vi "CalcOctaves.vi"(11 "Energy":cluster{"x0":dbl, "df":dbl, dbl[]}[](graph)) -> (1 "XY Graph":cluster{dbl[], dbl[]}[](graph), 2 "Prediction":dbl[](array[numeric]), 3 "Peak Freq":dbl[](array[numeric]))   [LabVIEW 2022 SP3]
uses:
  <vilib>/Analysis/NI_AAL_SigProc.lvlib
panel:
  out "Energy 2":cluster{"x0":dbl, "df":dbl, dbl[]}(graph)
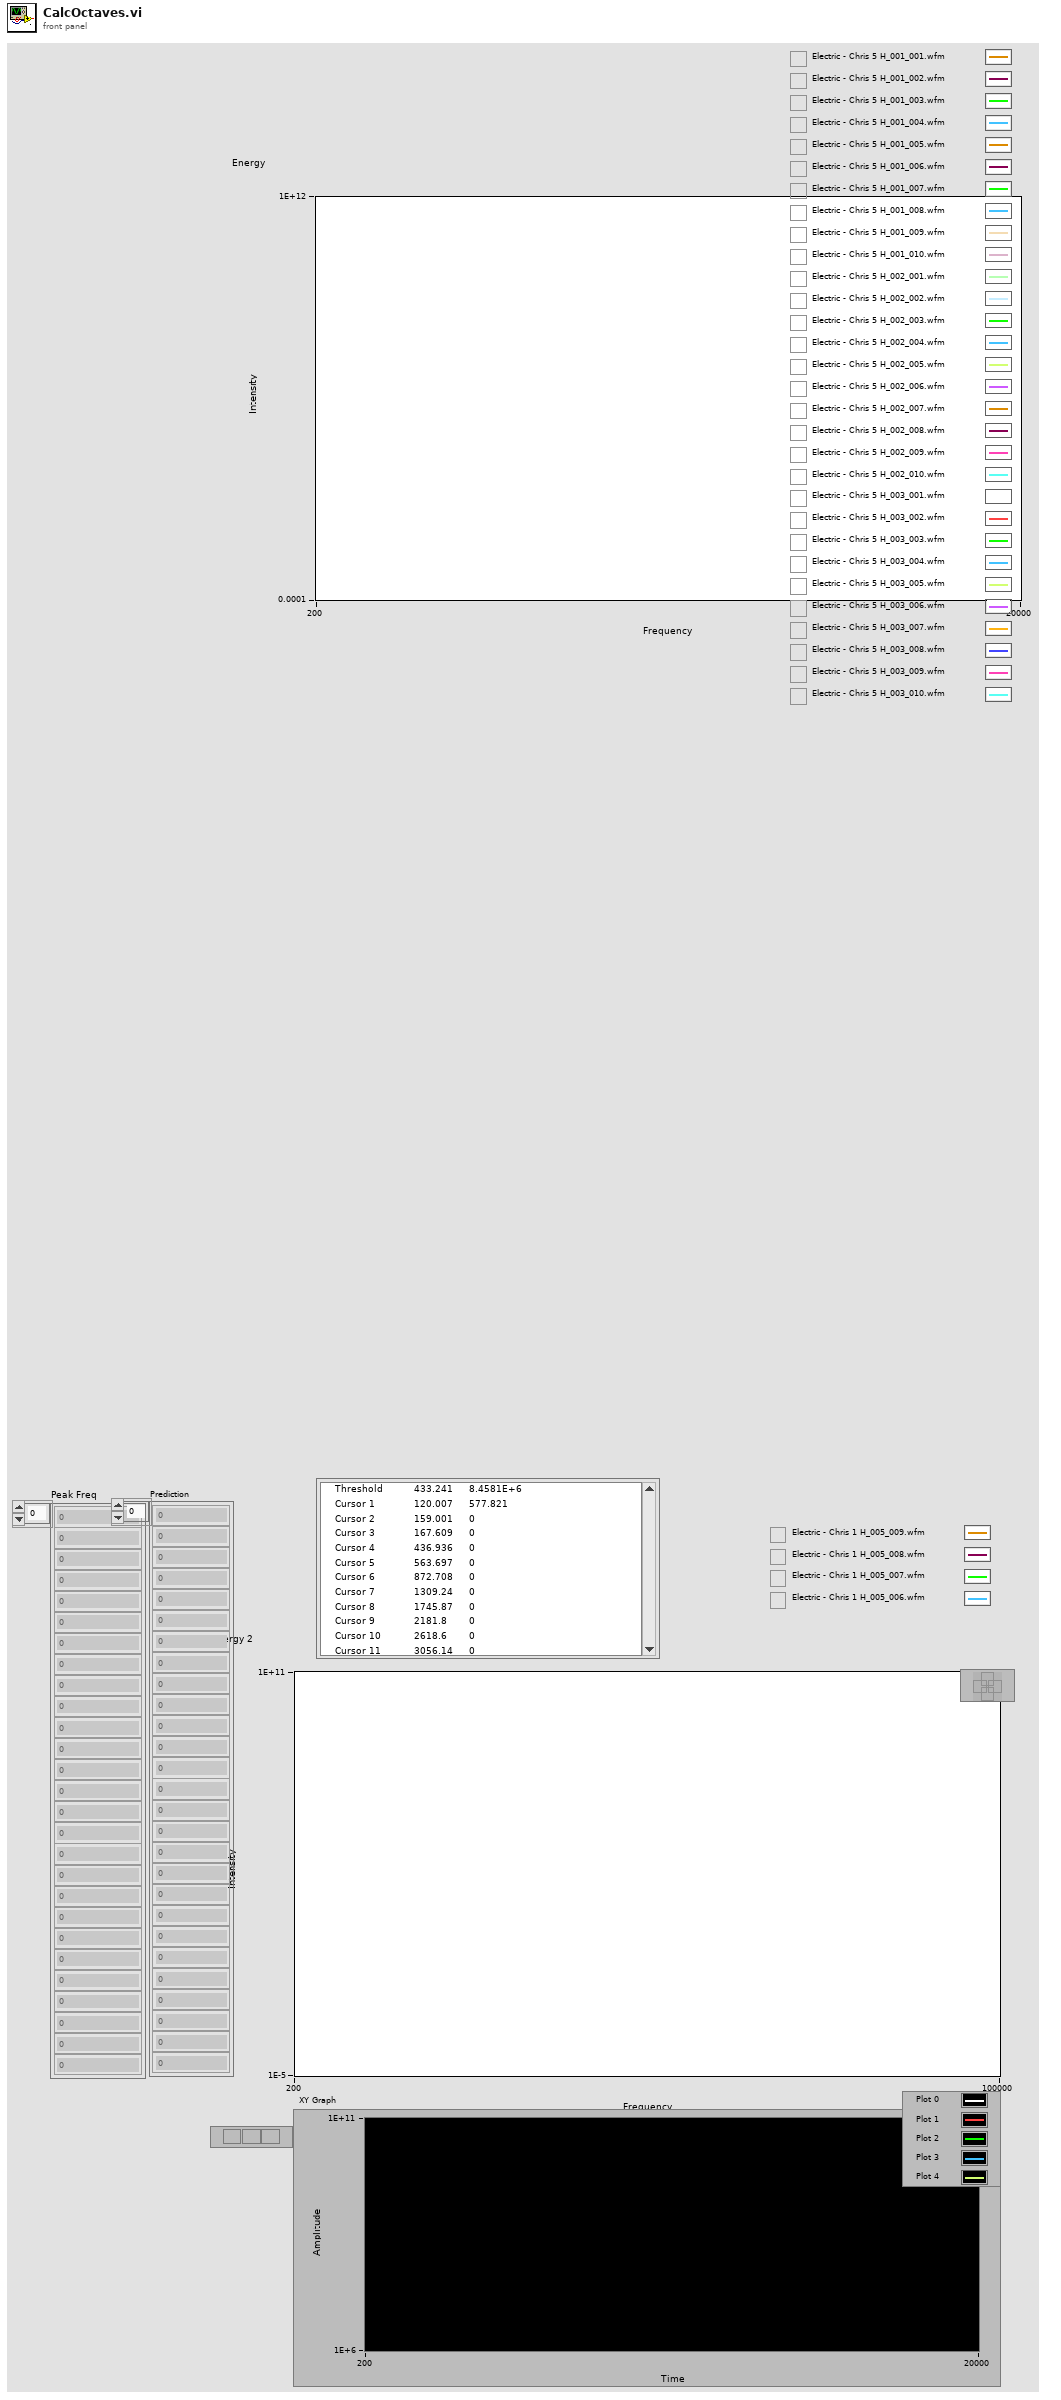
[diagram p1: front panel]
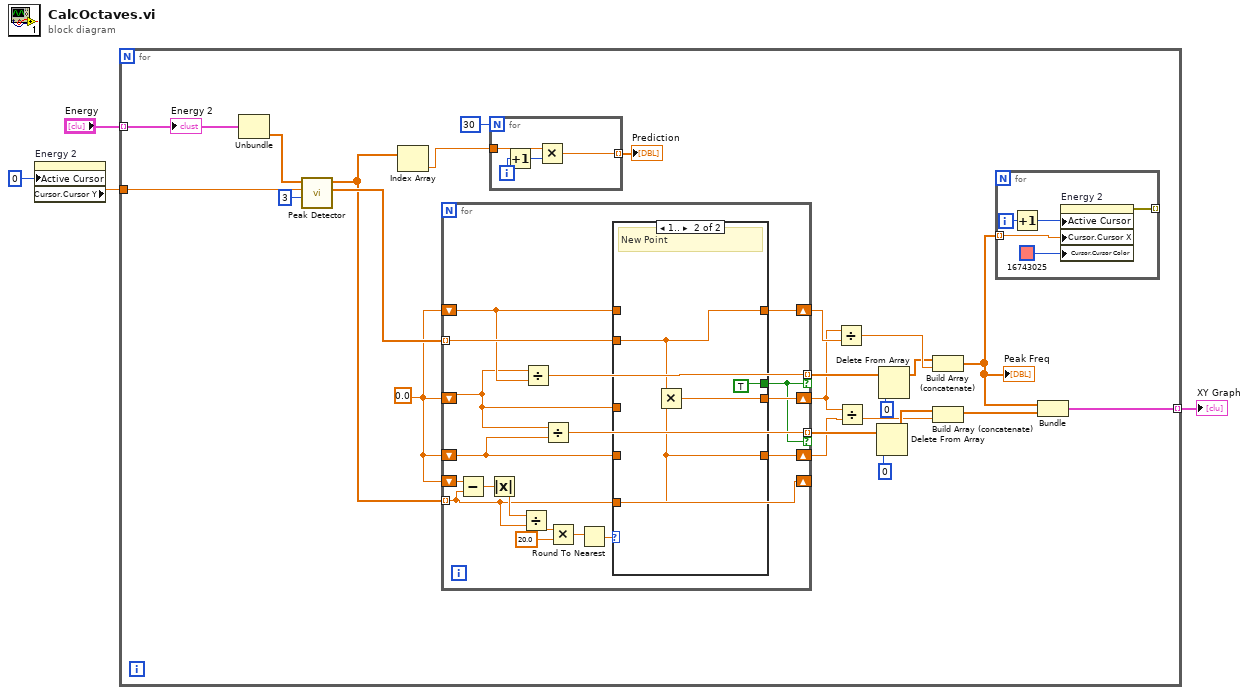
[diagram p0: block diagram]
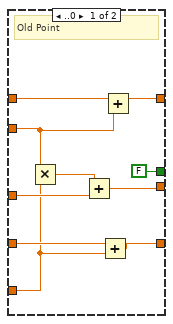
[diagram p2: hidden frame]
diagram:
  n1 = property on="Energy 2" class="WFGraph (strict)"("Active Cursor"=u32 0) -> ("Cursor.Cursor Y"=w3:dbl)  [unwired: 2 in, 2 out]
  n2 = for {
    tunnel: w3 -> [w27]
    tunnel: [w8] -> w2 mode=indexing
    tunnel: "Energy" -> [w5] mode=indexing
    w15 = 0.0
    n3 = Unbundle(w5) -> (w28:dbl[])  [unwired: 2 out]
    n4 = call <vilib>:"Peak Detector.vi"("width"=3, "threshold"=w27, "X"=w28) -> ("Amplitudes"=w24:dbl[], "Locations"=w20:dbl[])  [unwired: 4 in, 3 out]
    n5 = Index Array(array=w20) -> (element=w19:dbl)  [unwired: 1 in]
    n6 = for {
      tunnel: w20 -> [w43] mode=indexing
      shift-right: [w43] -> _
      shift-left: w15 -> [w50]
      shift-right: [w41] -> w12
      shift-left: w15 -> [w36]
      tunnel: [w42] -> w26 mode=indexing if=w33
      shift-right: [w39] -> w23
      shift-left: w15 -> [w38]
      tunnel: w24 -> [w40] mode=indexing
      shift-right: [w37] -> w11
      shift-left: w15 -> [w35]
      tunnel: [w34] -> w13 mode=indexing if=w33
      n7 = Subtract(x=w50, y=w43) -> (x-y=w49:dbl)
      n8 = Absolute Value(x=w49) -> (abs(x)=w48:dbl)
      n9 = Divide(x=w48, y=w43) -> (x/y=w47:dbl)
      n10 = Divide(x=w36, y=w38) -> (x/y=w42:dbl)
      n11 = Divide(x=w36, y=w35) -> (x/y=w34:dbl)
      n12 = Multiply(x=w47, y=20.0) -> (x*y=w45:dbl)
      n13 = Round To Nearest(number=w45) -> (nearest integer value=w44:dbl)
      n14 = case shown="1.." w44 {
        tunnel: w43 -> [w52 w61]
        tunnel: w36 -> [w57 _]
        tunnel: [w54 w63] -> w41
        tunnel: [FALSE TRUE] -> w33
        tunnel: w38 -> [w59 _]
        tunnel: [w58 w62] -> w39
        tunnel: w40 -> [w55 w62]
        tunnel: w35 -> [w53 _]
        tunnel: [w51 w61] -> w37
        frame ..0 {
          # "Old Point"
          n15 = Multiply(x=w55, y=w52) -> (x*y=w56:dbl)
          n16 = Add(x=w56, y=w57) -> (x+y=w54:dbl)
          n17 = Add(x=w53, y=w52) -> (x+y=w51:dbl)
          n18 = Add(x=w59, y=w55) -> (x+y=w58:dbl)
        }
        frame 1.. {
          # "New Point"
          n19 = Multiply(x=w62, y=w61) -> (x*y=w63:dbl)
        }
      }
    }
    n20 = for {
      N: 30 -> [_]
      tunnel: w19 -> [w32]
      tunnel: [w29] -> w18 mode=indexing
      i -> [w31]
      n21 = Increment(x=w31) -> (x+1=w30:i32)
      n22 = Multiply(x=w32, y=w30) -> (x*y=w29:dbl)
    }
    "Prediction" <- w18
    n23 = Divide(x=w12, y=w23) -> (x/y=w22:dbl)
    n24 = Divide(x=w12, y=w11) -> (x/y=w9:dbl)
    n25 = Delete From Array(array=w13, index=0) -> (array with subset deleted=w10:dbl[])  [unwired: 1 in, 1 out]
    n26 = Delete From Array(array=w26, index=0) -> (array with subset deleted=w21:dbl[])  [unwired: 1 in, 1 out]
    n27 = Build Array (concatenate)(w21, w22) -> (w7:dbl[])
    "Peak Freq" <- w7
    n28 = Build Array (concatenate)(w10, w9) -> (w6:dbl[])
    n29 = for {
      tunnel: w7 -> [w69] mode=indexing
      tunnel: [w65] -> _ mode=indexing
      i -> [w68]
      n30 = Increment(x=w68) -> (x+1=w67:i32)
      n31 = property on="Energy 2" class="WFGraph (strict)"("Active Cursor"=w67, "Cursor.Cursor X"=w69, "Cursor.Cursor Color"=u32 16743025) -> (error out=w65:errorcluster)  [unwired: 2 in, 1 out]
    }
    n32 = Bundle(w7, w6) -> (w8:cluster{dbl[], dbl[]})  [unwired: 1 in]
    "Energy 2" <- w5
  }
  "XY Graph" <- w2
